vi "Lesson3 - State Machine.vi"() -> ()   [LabVIEW 2013]
panel:
  out "is there error? 2":string
  out "Numeric Indicator 3":i32
  out "error out 2":errorcluster
  in  "Enum 2":enum16{"Hello", "You're Ewlcome", "Goodbye"}(ring)
  out "is there error?":string
  out "error out":errorcluster
  in  "Numeric":i32
  out "Numeric Indicator 2":i32
  out "Numeric Indicator":i32
  in  "String":string="True"
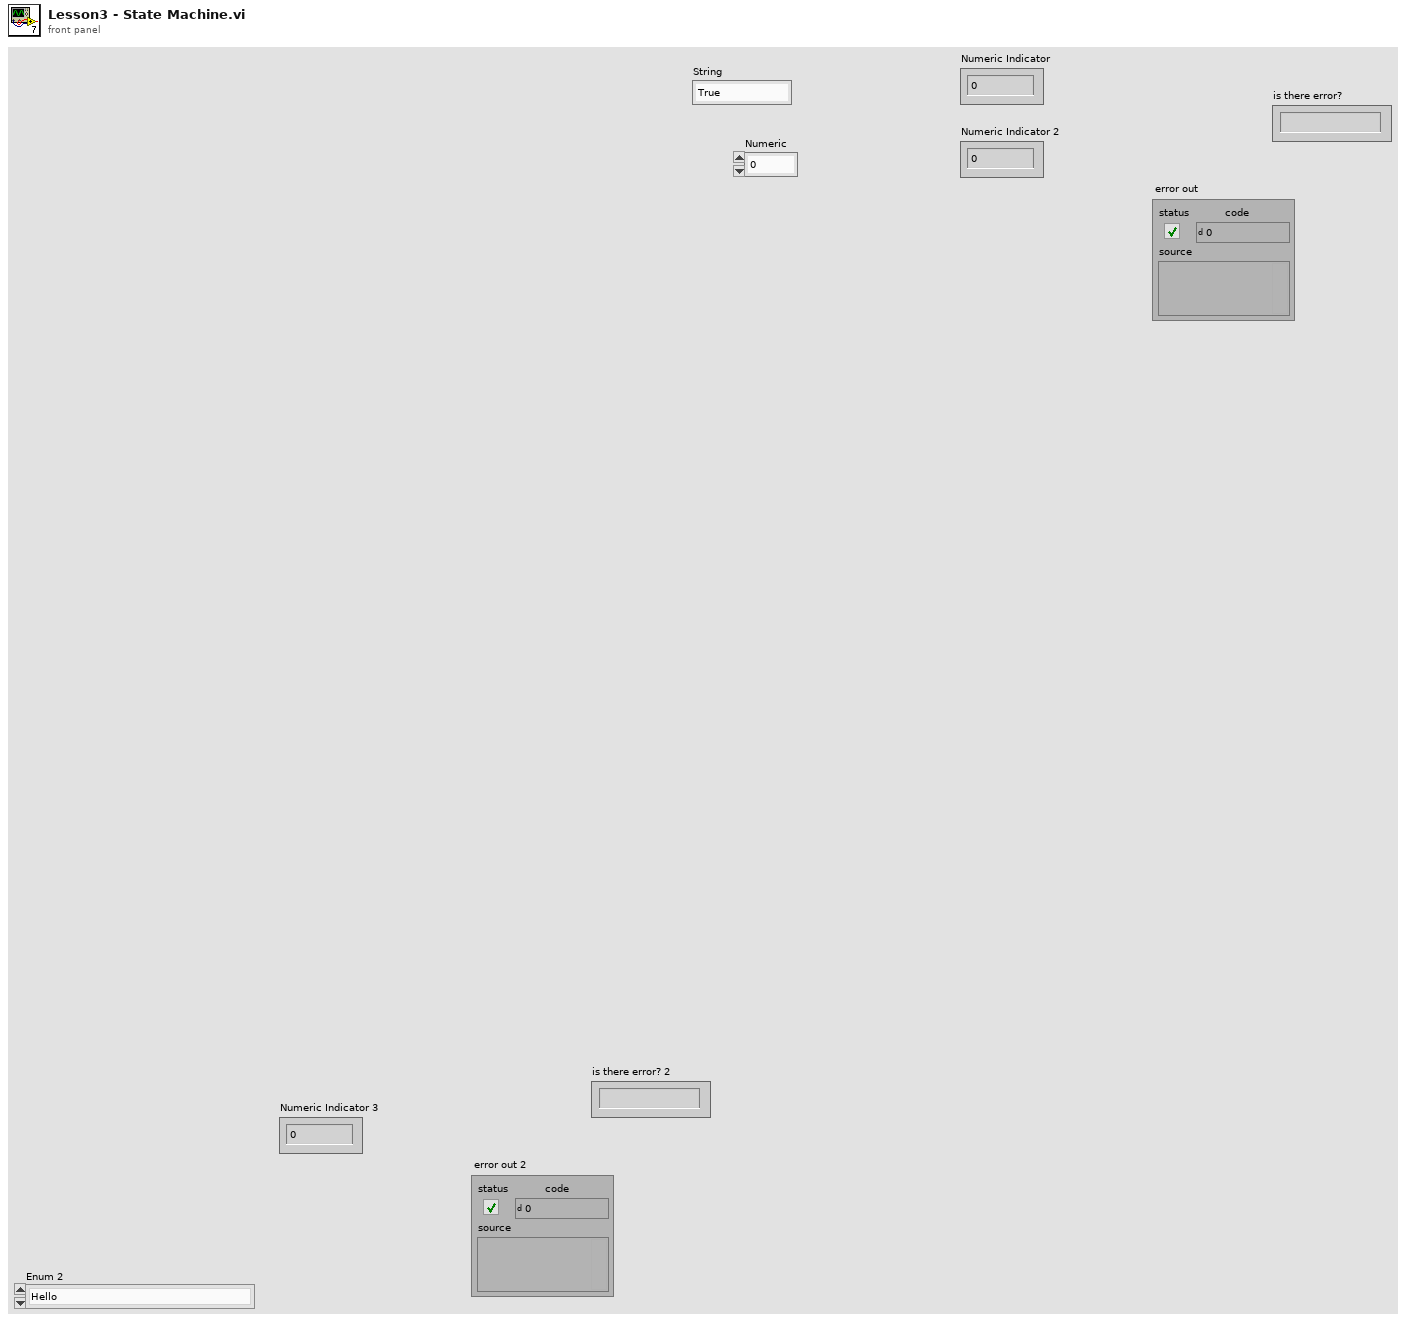
[diagram p1: front panel]
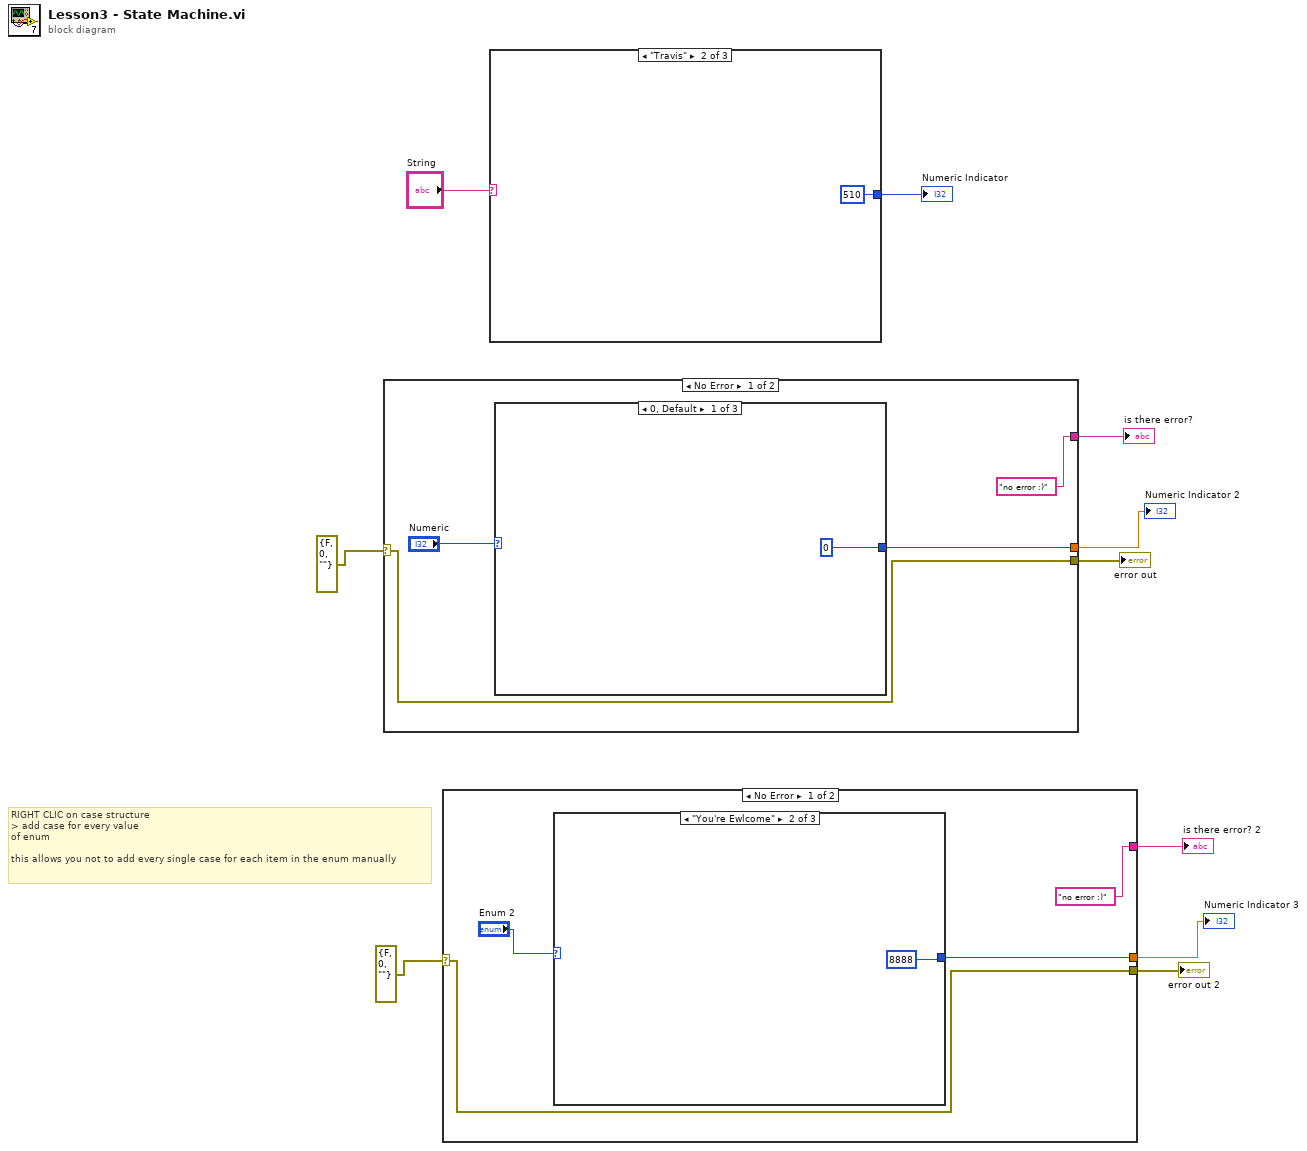
[diagram p0: block diagram]
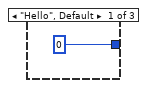
[diagram p2: hidden frame]
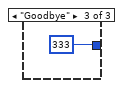
[diagram p3: hidden frame]
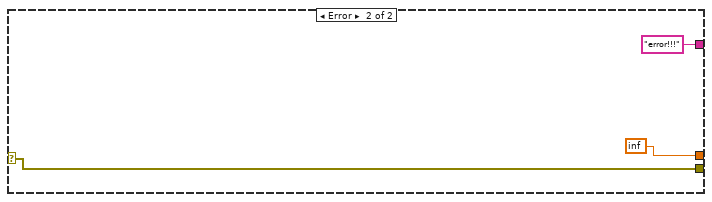
[diagram p4: hidden frame]
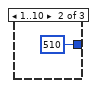
[diagram p5: hidden frame]
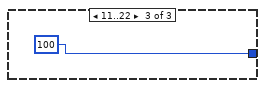
[diagram p6: hidden frame]
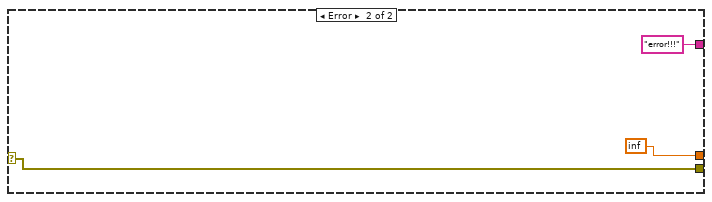
[diagram p7: hidden frame]
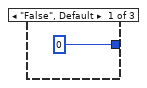
[diagram p8: hidden frame]
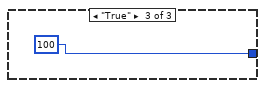
[diagram p9: hidden frame]
diagram:
  # "RIGHT CLIC on case structure\n> add case for every value\nof enum\n\nthis allows you not to add every single case for each item in the enum manually"
  n1 = case shown="No Error" errorcluster {"status"=FALSE, "code"=0, "source"=""} ("error constant") {
    selector: errorcluster {"status"=FALSE, "code"=0, "source"=""} ("error constant") -> [w13 w20]
    tunnel: [w13 w20] -> w7
    tunnel: [w12 inf] -> w6
    tunnel: ["no error :)" "error!!!"] -> w5
    frame No Error {
      n2 = case shown="0, Default" "Numeric" {
        tunnel: [0 ("Numeric") 510 ("Numeric") 100] -> w12
        frame 0, Default {
        }
        frame 1..10 {
        }
        frame 11..22 {
        }
      }
    }
    frame Error {
    }
  }
  "error out" <- w7
  "Numeric Indicator 2" <- w6
  "is there error?" <- w5
  n3 = case shown="No Error" errorcluster {"status"=FALSE, "code"=0, "source"=""} ("error constant") {
    selector: errorcluster {"status"=FALSE, "code"=0, "source"=""} ("error constant") -> [w24 w30]
    tunnel: [w24 w30] -> w3
    tunnel: [w23 inf] -> w2
    tunnel: ["no error :)" "error!!!"] -> w1
    frame No Error {
      n4 = case shown="\"You're Ewlcome\"" "Enum 2" {
        tunnel: [0 ("Numeric") 8888 333] -> w23
        frame "Hello", Default {
        }
        frame "You're Ewlcome" {
        }
        frame "Goodbye" {
        }
      }
    }
    frame Error {
    }
  }
  "error out 2" <- w3
  "Numeric Indicator 3" <- w2
  "is there error? 2" <- w1
  n5 = case shown="\"Travis\"" "String" {
    tunnel: [0 ("Numeric") 510 ("Numeric") 100] -> w9
    frame "False", Default {
    }
    frame "Travis" {
    }
    frame "True" {
    }
  }
  "Numeric Indicator" <- w9
